vi "rqcAlice SPI (FPGA).vi"(0 "data in":u32, 9 "write":bool) -> (4 "data":bool, 6 "we":bool, 8 "clk":bool)   [LabVIEW 2018]
uses:
  Custom Controls/Pseudo SPI/rqcAlice SPI state.ctl
  Custom Controls/Pseudo SPI/rqcAlice PS states.ctl
panel:
  in  "MSB first":bool=TRUE
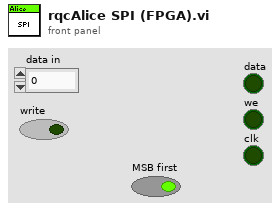
[diagram p1: front panel]
types:
  T1 = typedef "rqcAlice SPI state.ctl" = cluster{"data":bool[], "state":T2, "spi.data":bool, "spi.we":bool, "spi.clk":bool, "bits sent":u8}
  T2 = typedef "rqcAlice PS states.ctl" = enum16{"idle", "send"}
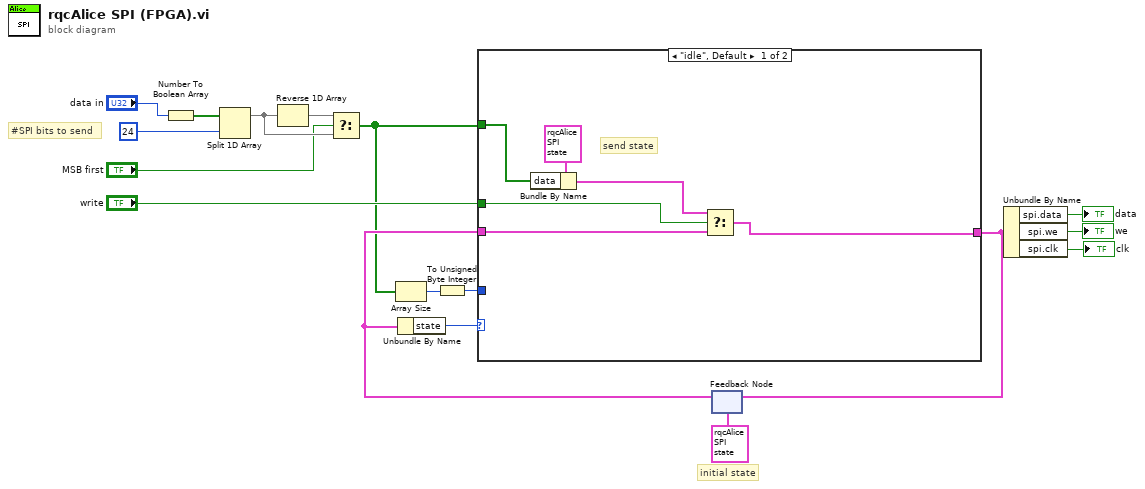
[diagram p0: block diagram]
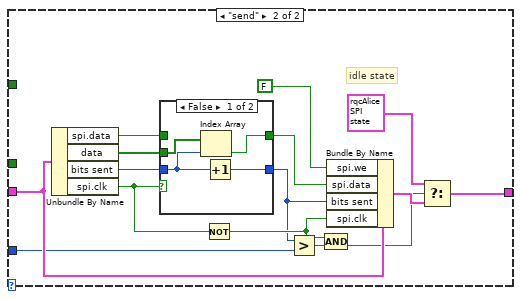
[diagram p2: hidden frame]
diagram:
  # "initial state"
  # "#SPI bits to send"
  n1 = Number To Boolean Array(number="data in") -> (Boolean array=w16:bool[])
  n2 = Split 1D Array(array=w16, index=u8 24) -> (first subarray=w15:bool[])  [unwired: 1 out]
  n3 = Reverse 1D Array(array=w15) -> (reversed array=w4:bool[])
  n4 = Select(t=w4, s="MSB first", f=w15) -> (s? t:f=w1:bool[])
  n5 = Array Size(array=w1) -> (size(s)=w3:i32)
  n6 = To Unsigned Byte Integer(number=w3) -> (unsigned 8bit integer=w2:u8)
  n7 = feedback #1(T1 {"data"=[FALSE, FALSE, FALSE, FALSE, FALSE, FALSE, FALSE, FALSE, FALSE, FALSE, FALSE, FALSE, FALSE, FALSE, FALSE, FALSE, FALSE, FALSE, FALSE, FALSE, FALSE, FALSE, FALSE, FALSE], "state"=enum."idle", "spi.data"=FALSE, "spi.we"=TRUE, "spi.clk"=FALSE, "bits sent"=0} ("PS state cluster")) -> (w10:T1)
  n8 = Unbundle By Name(w10) -> ("state"=w11:T2)
  n9 = case shown="\"idle\", Default" w11 {
    tunnel: w2 -> [_ w25]
    tunnel: w1 -> [w21 _]
    tunnel: "write" -> [w18 _]
    tunnel: [w19 w31] -> w9
    tunnel: w10 -> [w20 w38]
    frame "idle", Default {
      # "send state"
      n10 = Bundle By Name(cluster=T1 {"data"=[FALSE, FALSE, FALSE, FALSE, FALSE, FALSE, FALSE, FALSE, FALSE, FALSE, FALSE, FALSE, FALSE, FALSE, FALSE, FALSE, FALSE, FALSE, FALSE, FALSE, FALSE, FALSE, FALSE, FALSE], "state"=enum."send", "spi.data"=FALSE, "spi.we"=TRUE, "spi.clk"=FALSE, "bits sent"=0} ("PS state cluster"), "data"=w21) -> (w23:T1)
      n11 = Select(t=w23, s=w18, f=w20) -> (s? t:f=w19:T1)
    }
    frame "send" {
      # "idle state"
      n12 = Unbundle By Name(w38) -> ("spi.data"=w35:bool, "data"=w37:bool[], "bits sent"=w36:u8, "spi.clk"=w33:bool)
      n13 = case shown="False" w33 {
        tunnel: w37 -> [w42 _]
        tunnel: w36 -> [w40 w43]
        tunnel: [w41 w44] -> w34
        tunnel: w35 -> [_ w44]
        tunnel: [w39 w43] -> w26
        frame False {
          n14 = Index Array(array=w42, index=w40) -> (element=w41:bool)
          n15 = Increment(x=w40) -> (x+1=w39:u8)
        }
        frame True {
        }
      }
      n16 = Not(x=w33) -> (.not. x?=w27:bool)
      n17 = Greater?(x=w26, y=w25) -> (0:w32:bool)
      n18 = Compound Arithmetic op=AND(w27, w32) -> (w28:bool)
      n19 = Bundle By Name(cluster=w38, "spi.we"=FALSE, "spi.data"=w34, "bits sent"=w26, "spi.clk"=w27) -> (w30:T1)
      n20 = Select(t=T1 {"data"=[FALSE, FALSE, FALSE, FALSE, FALSE, FALSE, FALSE, FALSE, FALSE, FALSE, FALSE, FALSE, FALSE, FALSE, FALSE, FALSE, FALSE, FALSE, FALSE, FALSE, FALSE, FALSE, FALSE, FALSE], "state"=enum."idle", "spi.data"=FALSE, "spi.we"=TRUE, "spi.clk"=FALSE, "bits sent"=0} ("PS state cluster"), s=w28, f=w30) -> (s? t:f=w31:T1)
    }
  }
  n21 = feedback-in #1(w9) -> ()
  n22 = Unbundle By Name(w9) -> ("spi.data"=→"data":bool, "spi.we"=→"we":bool, "spi.clk"=→"clk":bool)
